vi "LVITX Read Folder Index.vi"(11 "File or Folder Path":path) -> (3 "Array":path[](array[path]))   [LabVIEW 2013]
uses:
  <vilib>/Utility/file.llb/Read From Spreadsheet File (string).vi
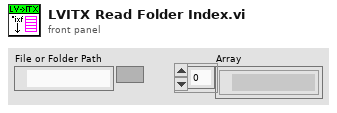
[diagram p1: front panel]
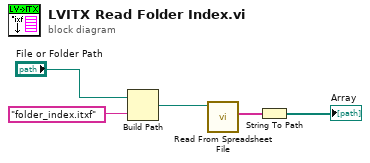
[diagram p0: block diagram]
diagram:
  n1 = Build Path(base path="File or Folder Path", name or relative path="folder_index.itxf") -> (appended path=w3:path)
  n2 = call-poly <vilib>:"Read From Spreadsheet File.vi"("file path (dialog if empty)"=w3) -> ("first row"=w5:string[])  [unwired: 6 in, 4 out]
  n3 = String To Path(string=w5) -> (path=→"Array":path[])
